vi "SQL.TestResult.vi"(0 "FINDstatus":bool=TRUE, 1 "FINDnumber":bool=TRUE, 2 "FINDtime":bool=TRUE, 3 "FINDdata":bool=TRUE, 6 "error in (no error)":errorcluster, 7 "Folder Path":path caption="文件夹路径", 8 "status":string, 9 "serialnumber":string, 10 "time":string, 11 "date":string) -> (4 "error out":errorcluster, 5 "SQL Results":string[][](table)=[["1.Audio RX", "91.081303", "2.Audio TX", "0.095270", "20121122", "13:32:50", "1170000000689", "PASS"], ["1.Audio RX", "91.143105", "2.Audio TX", "0.095494", "20121122", "13:39:33", "1170000000689", "PASS"], ["1.Audio RX", "91.991153", "2.Audio TX", "0.100831", "20121122", "13:54:04", "1111111111111", "PASS"], ["1.Audio RX", "91.857442", "2.Audio TX", "0.105589", "20121122", "13:56:23", "1172000000041", "PASS"], ["1.Audio RX", "92.085102", "2.Audio TX", "0.101190", "20121122", "13:57:37", "1172000000027", "PASS"], ["1.Audio RX", "91.878361", "2.Audio TX", "0.100191", "20121122", "13:59:11", "1172000000362", "PASS"], ["1.Audio RX", "92.029742", "2.Audio TX", "0.098333", "20121122", "14:02:06", "1172000000287", "PASS"], ["1.Audio RX", "91.480339", "2.Audio TX", "0.101565", "20121122", "14:04:55", "1170000000436", "PASS"], ["1.Audio RX", "91.969090", "2.Audio TX", "0.101169", "20121122", "14:06:27", "1172000000171", "PASS"], ["1.Audio RX", "92.221462", "2.Audio TX", "0.099581", "20121122", "14:09:34", "1172000000034", "PASS"], ["1.Audio RX", "91.987652", "2.Audio TX", "0.098084", "20121122", "14:11:36", "1172000000317", "PASS"], ["1.Audio RX", "92.074553", "2.Audio TX", "0.099366", "20121122", "14:13:21", "1172000000263", "PASS"], ["1.Audio RX", "92.132843", "2.Audio TX", "0.098619", "20121122", "14:14:51", "1172000000492", "PASS"], ["1.Audio RX", "92.082562", "2.Audio TX", "0.099291", "20121122", "14:16:15", "1172000000010", "PASS"], ["1.Audio RX", "91.950055", "2.Audio TX", "0.100073", "20121122", "14:17:31", "1172000000041", "PASS"], ["1.Audio RX", "92.103586", "2.Audio TX", "0.100658", "20121122", "14:28:07", "0000000000000", "PASS"], ["1.Audio RX", "92.130135", "2.Audio TX", "0.099393", "20121122", "14:31:21", "1172000000331", "PASS"], ["1.Audio RX", "92.260601", "2.Audio TX", "0.099085", "20121122", "14:33:09", "1172000000416", "PASS"], ["1.Audio RX", "91.917260", "2.Audio TX", "0.099118", "20121122", "14:34:45", "1172000000294", "PASS"], ["1.Audio RX", "91.905751", "2.Audio TX", "0.097974", "20121122", "14:36:10", "1172000000423", "PASS"], ["1.Audio RX", "92.133605", "2.Audio TX", "0.097918", "20121122", "14:37:41", "1172000000119", "PASS"], ["1.Audio RX", "92.096734", "2.Audio TX", "0.102493", "20121122", "14:40:09", "1172000000508", "PASS"], ["1.Audio RX", "92.042766", "2.Audio TX", "0.097988", "20121122", "14:41:47", "1172000000157", "PASS"], ["1.Audio RX", "92.072530", "2.Audio TX", "0.098405", "20121122", "14:42:41", "1172000000157", "PASS"], ["1.Audio RX", "91.988608", "2.Audio TX", "0.100953", "20121122", "14:45:30", "1172000000164", "PASS"], ["1.Audio RX", "92.115288", "2.Audio TX", "0.099866", "20121122", "14:46:43", "1172000000379", "PASS"], ["1.Audio RX", "91.931552", "2.Audio TX", "0.098401", "20121122", "14:48:07", "1172000000201", "PASS"], ["1.Audio RX", "92.141466", "2.Audio TX", "0.102419", "20121122", "14:49:20", "1172000000324", "PASS"], ["1.Audio RX", "91.932576", "2.Audio TX", "0.099878", "20121122", "14:51:57", "1172000000355", "PASS"], ["1.Audio RX", "92.147045", "2.Audio TX", "0.096185", "20121122", "14:54:23", "1172000000133", "PASS"], ["1.Audio RX", "92.010262", "2.Audio TX", "0.097653", "20121122", "14:55:55", "1172000000270", "PASS"], ["1.Audio RX", "92.200920", "2.Audio TX", "0.099317", "20121122", "14:57:32", "1172000000065", "PASS"], ["1.Audio RX", "92.066286", "2.Audio RX", "91.980270", "20121122", "15:11:29", "", "PASS"], ["1.Audio RX", "92.152783", "2.Audio RX", "92.048697", "20121122", "15:14:00", "", "PASS"], ["1.Audio RX", "92.058673", "2.Audio TX", "0.099819", "20121122", "15:54:48", "1170000000689", "PASS"], ["1.Audio RX", "91.953046", "2.Audio TX", "0.099171", "20121122", "15:58:55", "1170000000436", "PASS"]])   [LabVIEW 2012, in "Lib_UEL.ATE.lvlib" / "Lib_SQL.lvlib"]
uses:
  Lib_SQL.lvlib
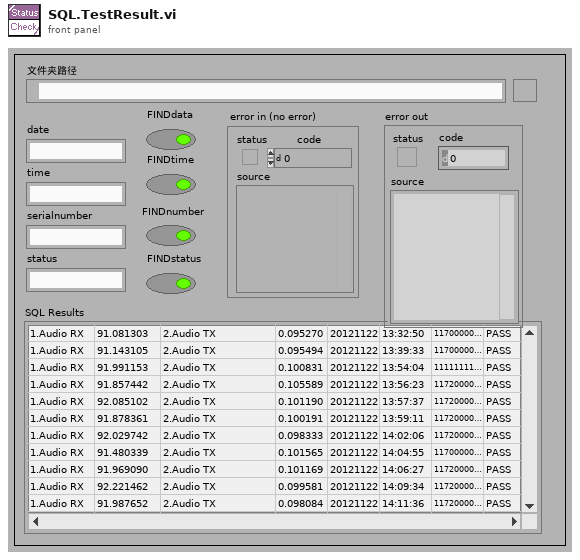
[diagram p1: front panel]
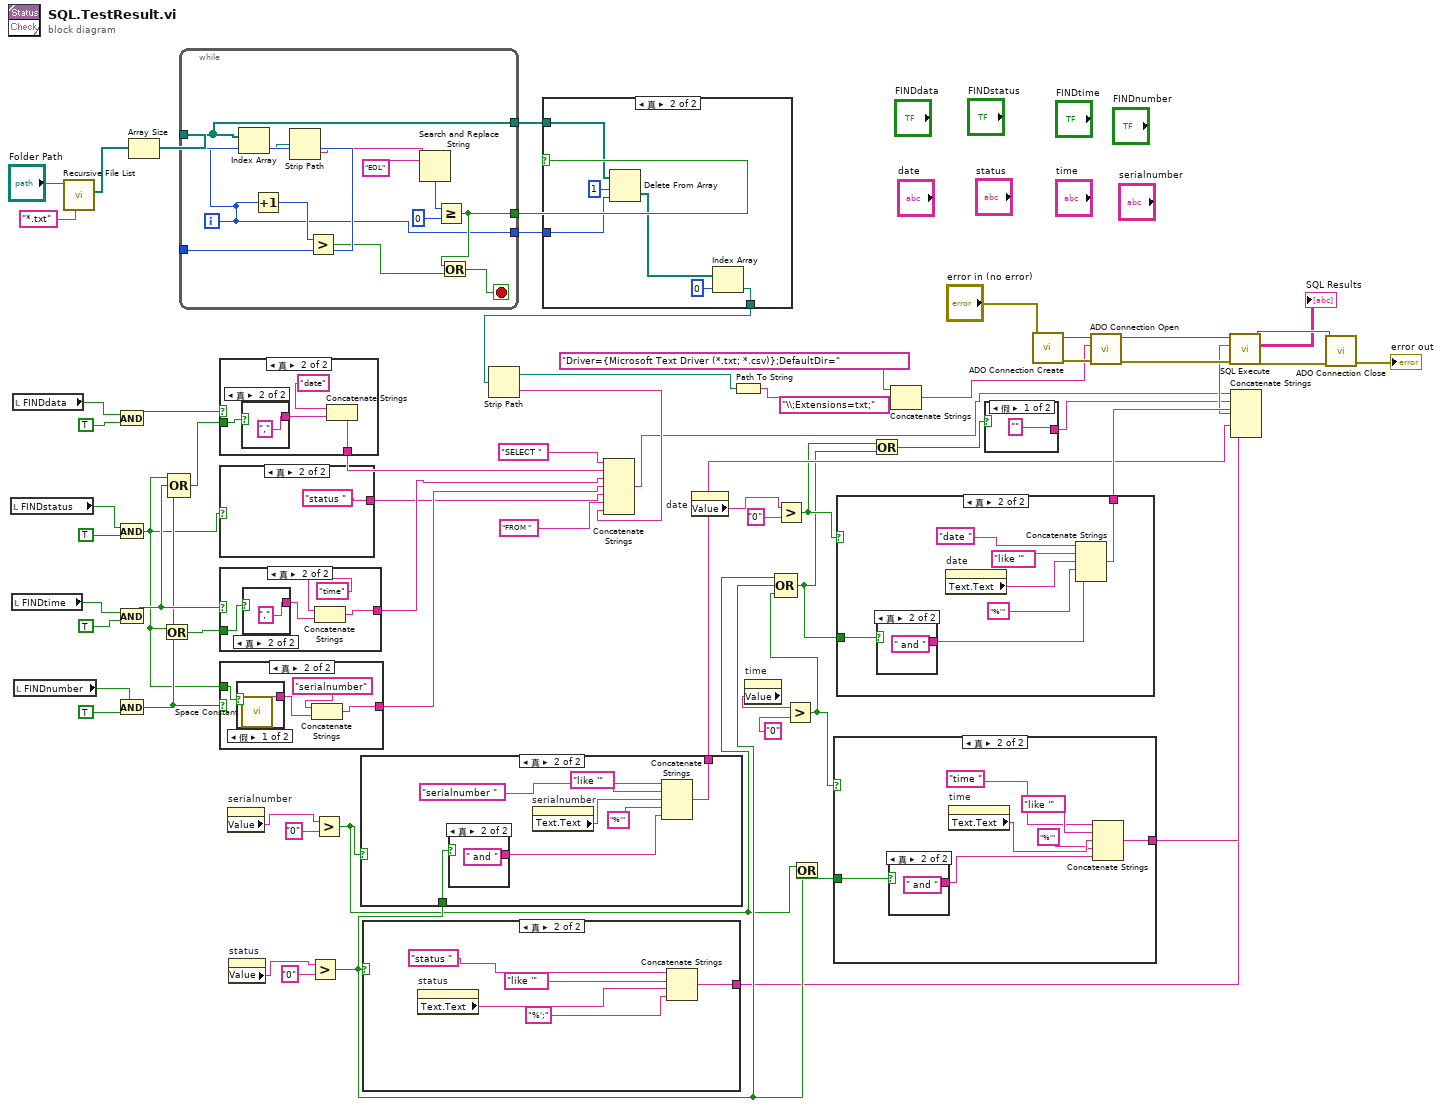
[diagram p0: block diagram]
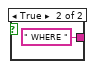
[diagram p2: hidden frame]
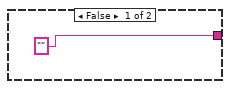
[diagram p4: hidden frame]
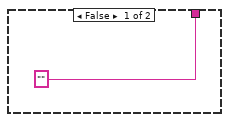
[diagram p5: hidden frame]
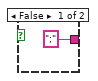
[diagram p6: hidden frame]
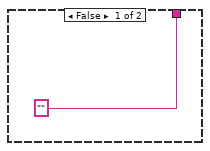
[diagram p7: hidden frame]
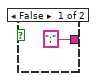
[diagram p8: hidden frame]
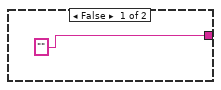
[diagram p9: hidden frame]
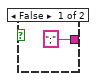
[diagram p10: hidden frame]
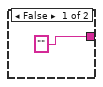
[diagram p11: hidden frame]
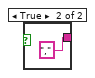
[diagram p12: hidden frame]
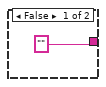
[diagram p13: hidden frame]
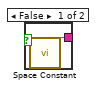
[diagram p14: hidden frame]
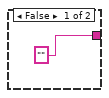
[diagram p15: hidden frame]
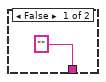
[diagram p16: hidden frame]
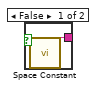
[diagram p17: hidden frame]
diagram:
  n1 = local read "FINDstatus"() -> (w56:bool)
  n2 = local read "FINDtime"() -> (w54:bool)
  n3 = local read "FINDdata"() -> (w59:bool)
  n4 = local read "FINDnumber"() -> (w52:bool)
  n5 = call <vilib>:"Recursive File List.vi"("pattern"="*.txt", "Folder Path"="Folder Path") -> ("All Files in Dir"=w11:path[])  [unwired: 5 in, 4 out]
  n6 = And(x=w59, y=TRUE) -> (x .and. y?=w58:bool)
  n7 = And(x=w56, y=TRUE) -> (x .and. y?=w43:bool)
  n8 = And(x=w54, y=TRUE) -> (x .and. y?=w47:bool)
  n9 = And(x=w52, y=TRUE) -> (x .and. y?=w44:bool)
  n10 = Array Size(array=w11) -> (size(s)=w9:i32)
  n11 = Or(x=w43, y=w44) -> (x .or. y?=w45:bool)
  n12 = Compound Arithmetic op=OR(w43, w47, w44) -> (w46:bool)
  n13 = while {
    tunnel: w11 -> [w69]
    tunnel: [w69] -> w10
    tunnel: w9 -> [w68]
    tunnel: [w67] -> w8
    tunnel: [w66] -> w7
    i -> [w66]
    stop <- w70 stop-if-true
    n14 = Index Array(array=w69, index=w66) -> (element=w72:path)
    n15 = Increment(x=w66) -> (x+1=w76:i32)
    n16 = Strip Path(path=w72) -> (name=w71:string)  [unwired: 1 out]
    n17 = Greater?(x=w76, y=w68) -> (0:w73:bool)
    n18 = Search and Replace String(input string=w71, search string="EOL" ("搜索字符串")) -> (offset past replacement=w75:i32)  [unwired: 6 in, 3 out]
    n19 = Greater Or Equal?(x=w75, y=0) -> (x >= y?=w67:bool)
    n20 = Or(x=w67, y=w73) -> (x .or. y?=w70:bool)
  }
  n21 = case shown="真" w58 {
    tunnel: ["" w80] -> w51
    tunnel: w46 -> [_ w79]
    frame False {
    }
    frame True {
      n22 = case shown="真" w79 {
        tunnel: [w83 ","] -> w81
        frame False {
          n23 = call <vilib>:"Space Constant.vi"() -> ("String"=w83:string)
        }
        frame True {
        }
      }
      n24 = Concatenate Strings("date", w81) -> (w80:string)
    }
  }
  n25 = case shown="真" w43 {
    tunnel: ["" "status "] -> w48
    frame False {
    }
    frame True {
    }
  }
  n26 = case shown="真" w47 {
    tunnel: ["" w89] -> w50
    tunnel: w45 -> [_ w91]
    frame False {
    }
    frame True {
      n27 = case shown="真" w91 {
        tunnel: [w92 ","] -> w90
        frame False {
          n28 = call <vilib>:"Space Constant.vi"() -> ("String"=w92:string)
        }
        frame True {
        }
      }
      n29 = Concatenate Strings("time", w90) -> (w89:string)
    }
  }
  n30 = case shown="真" w44 {
    tunnel: ["" w95] -> w49
    tunnel: w43 -> [_ w98]
    frame False {
    }
    frame True {
      n31 = case shown="假" w98 {
        tunnel: [w99 ","] -> w97
        frame False {
          n32 = call <vilib>:"Space Constant.vi"() -> ("String"=w99:string)
        }
        frame True {
        }
      }
      n33 = Concatenate Strings("serialnumber", w97) -> (w95:string)
    }
  }
  n34 = property on="serialnumber" class="Str"() -> ("Value"=w34:string)  [unwired: 2 in, 2 out]
  n35 = property on="status" class="Str"() -> ("Value"=w33:string)  [unwired: 2 in, 2 out]
  n36 = Greater?(x=w33, y="0") -> (0:w30:bool)
  n37 = Greater?(x=w34, y="0") -> (0:w29:bool)
  n38 = case shown="真" w29 {
    tunnel: w30 -> [_ w104]
    tunnel: ["" w103] -> w26
    frame False {
    }
    frame True {
      n39 = case shown="真" w104 {
        tunnel: [";" " and "] -> w105
        frame False {
        }
        frame True {
        }
      }
      n40 = property on="serialnumber" class="Str"() -> ("Text.Text"=w107:string)  [unwired: 2 in, 2 out]
      n41 = Concatenate Strings("serialnumber ", "like '", w107, "%'", w105) -> (w103:string)
    }
  }
  n42 = case shown="真" w30 {
    tunnel: ["" w113] -> w25
    frame False {
    }
    frame True {
      n43 = property on="status" class="Str"() -> ("Text.Text"=w115:string)  [unwired: 2 in, 2 out]
      n44 = Concatenate Strings("status ", "like '", w115, "%';") -> (w113:string)
    }
  }
  n45 = case shown="真" w8 {
    tunnel: w10 -> [_ w119]
    tunnel: w7 -> [_ w118]
    tunnel: [_ w117] -> w6
    frame False {
    }
    frame True {
      n46 = Delete From Array(array=w119, length=1 ("长度"), index=w118) -> (deleted portion=w120:path[])  [unwired: 1 out]
      n47 = Index Array(array=w120, index=0 ("索引")) -> (element=w117:path)
    }
  }
  n48 = Strip Path(path=w6) -> (stripped path=w40:path, name=w63:string)
  n49 = Concatenate Strings("SELECT ", w51, w50, w49, w48, "FROM ", w63) -> (w5:string)
  n50 = property on="date" class="Str"() -> ("Value"=w35:string)  [unwired: 2 in, 2 out]
  n51 = Path To String(path=w40) -> (string=w41:string)
  n52 = property on="time" class="Str"() -> ("Value"=w62:string)  [unwired: 2 in, 2 out]
  n53 = Greater?(x=w35, y="0") -> (0:w3:bool)
  n54 = Greater?(x=w62, y="0") -> (0:w32:bool)
  n55 = Compound Arithmetic op=OR(w29, w30, w32) -> (w2:bool)
  n56 = Or(x=w29, y=w30) -> (x .or. y?=w31:bool)
  n57 = case shown="真" w32 {
    tunnel: w31 -> [_ w126]
    tunnel: ["" w125] -> w27
    frame False {
    }
    frame True {
      n58 = case shown="真" w126 {
        tunnel: [";" " and "] -> w127
        frame False {
        }
        frame True {
        }
      }
      n59 = property on="time" class="Str"() -> ("Text.Text"=w129:string)  [unwired: 2 in, 2 out]
      n60 = Concatenate Strings("time ", "like '", w129, "%'", w127) -> (w125:string)
    }
  }
  n61 = case shown="真" w3 {
    tunnel: w2 -> [_ w136]
    tunnel: ["" w135] -> w28
    frame False {
    }
    frame True {
      n62 = case shown="真" w136 {
        tunnel: [";" " and "] -> w137
        frame False {
        }
        frame True {
        }
      }
      n63 = property on="date" class="Str"() -> ("Text.Text"=w139:string)  [unwired: 2 in, 2 out]
      n64 = Concatenate Strings("date ", "like '", w139, "%'", w137) -> (w135:string)
    }
  }
  n65 = Or(x=w3, y=w2) -> (x .or. y?=w4:bool)
  n66 = Concatenate Strings("Driver={Microsoft Text Driver (*.txt; *.csv)};DefaultDir=", w41, "\\;Extensions=txt;" ("字符串")) -> (w15:string)
  n67 = case shown="假" w4 {
    tunnel: ["" " WHERE " ("字符串")] -> w1
    frame False {
    }
    frame True {
    }
  }
  n68 = call <userlib>:"ADO Connection Create.vi"("error in (no error)"="error in (no error)") -> ("error out"=w23:errorcluster, "ADODB._Connection Out"=w24:refnum<k7>)  [unwired: 9 in]
  n69 = call <userlib>:"ADO Connection Open.vi"("error in (no error)"=w23, "ConnectionString"=w15, "ADODB._Connection In"=w24) -> ("error out"=w21:errorcluster, "ADODB._Connection Out"=w22:refnum<k7>)  [unwired: 7 in]
  n70 = Concatenate Strings(w5, w1, w28, w27, w26, w25) -> (w14:string)
  n71 = call <userlib>:"SQL Execute.vi"("error in (no error)"=w21, "Command Text"=w14, "ADODB._Connection In"=w22) -> ("error out"=w20:errorcluster, "Data"=→"SQL Results":string[][], "ADODB._Connection Out"=w19:refnum<k7>)  [unwired: 5 in, 1 out]
  n72 = call <userlib>:"ADO Connection Close.vi"("error in (no error)"=w20, "ADODB._Connection In"=w19) -> ("error out"=→"error out":errorcluster)  [unwired: 8 in, 1 out]
